vi "test_Multiple Static Single Channel Command Messages using Trigger and Padding.vi"(8 "error in (no error)":errorcluster, 11 "TestCase in":refnum<class "Common System Tests.lvclass">) -> (0 "error out":errorcluster, 3 "TestCase out":refnum<class "Common System Tests.lvclass">)   [LabVIEW 2018, in "Common System Tests.lvclass"]
uses:
  Common System Tests.lvclass
  <vilib>/addons/_JKI Toolkits/VI Tester/TestCase.llb/TestCase.lvclass
  <vilib>/NI VeriStand/Execution/Workspace/NI_VS Workspace ExecutionAPI.lvlib
  <vilib>/NI VeriStand/Execution/Workspace/NI VeriStand - Set Single Channel Value.vi
  <vilib>/NI VeriStand/Execution/Workspace/NI VeriStand - Get Multiple Channel Values.vi
  C:/Program Files (x86)/National Instruments/LabVIEW 2019/vi.lib/addons/_JKI Toolkits/VI Tester/TestCase.llb/TestCase.lvclass
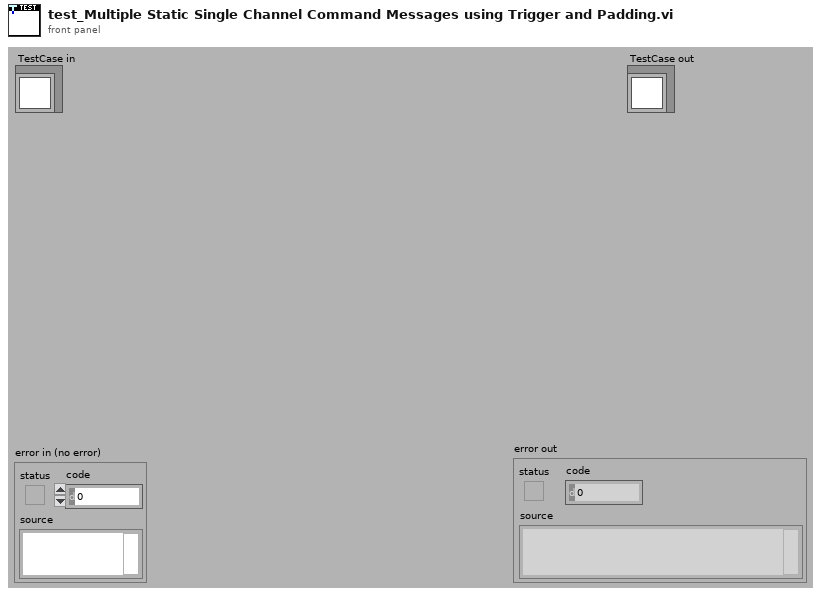
[diagram p1: front panel]
types:
  T1 = typedef "NI_VS Workspace ExecutionAPI.lvlib/WorkspaceAPI.ctl" = refnum<k24>
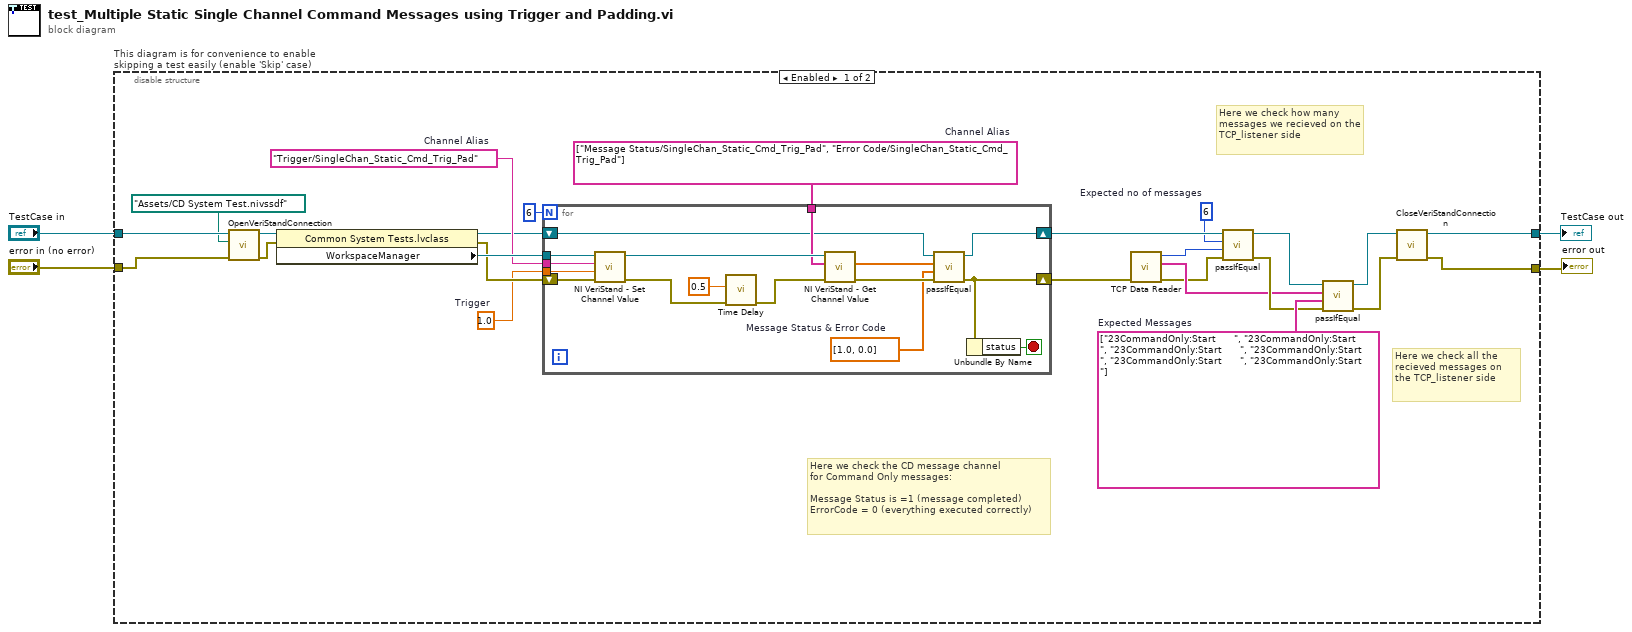
[diagram p0: block diagram]
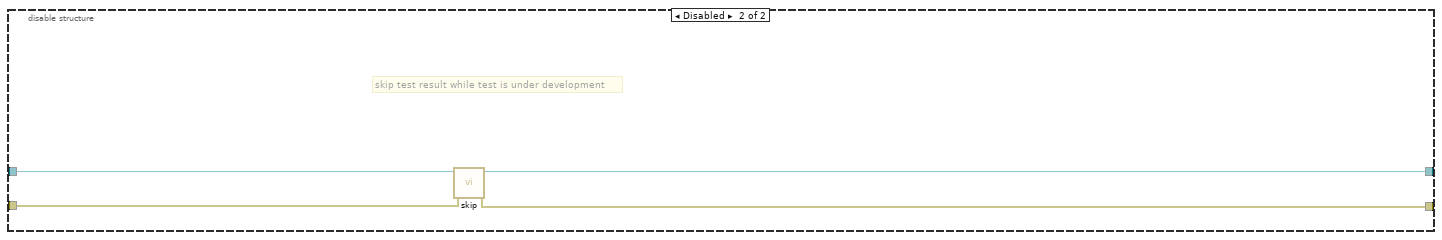
[diagram p2: hidden frame]
diagram:
  n1 = disable-structure "This diagram is for convenience to enable skipping a test easily (enable 'Skip' case)" shown="Enabled" {
    disable-tunnel: "TestCase in" -> [w27 w49]
    disable-tunnel: [w28 w47] -> w1
    disable-tunnel: [w29 w48] -> w3
    disable-tunnel: "error in (no error)" -> [w25 w46]
    frame Enabled {
      w11 = string[] ["23CommandOnly:Start      ", "23CommandOnly:Start      ", "23CommandOnly:Start      ", "23CommandOnly:Start      ", "23CommandOnly:Start      ", "23CommandOnly:Start      "]  # Expected Messages
      w13 = string[] ["Message Status/SingleChan_Static_Cmd_Trig_Pad", "Error Code/SingleChan_Static_Cmd_Trig_Pad"]  # Channel Alias
      w10 = 6  # Expected no of messages
      w19 = 1.0  # Trigger
      w20 = "Trigger/SingleChan_Static_Cmd_Trig_Pad"  # Channel Alias
      # "Here we check all the recieved messages on the TCP_listener side"
      # "Here we check how many messages we recieved on the TCP_listener side"
      # "Here we check the CD message channel\nfor Command Only messages:\n\nMessage Status is =1 (message completed)\nErrorCode = 0 (everything executed correctly)"
      n2 = call-dynamic "OpenVeriStandConnection.vi"("error in (no error)"=w25, "System Definition File"=path "Assets/CD System Test.nivssdf", "VeriStand Test Case in"=w27) -> ("error out"=w24:errorcluster, "VeriStand Test Case out"=w26:refnum<class "Common System Tests.lvclass">)  [unwired: 6 in, 1 out]
      n3 = property class="Common System Tests.lvclass"(reference=w26, error in=w24) -> (reference out=w17:refnum<class "Common System Tests.lvclass">, error out=w21:errorcluster, "WorkspaceManager"=w22:T1)
      n4 = for {
        N: 6 -> [_]
        tunnel: w22 -> [w45]
        tunnel: w20 -> [w43]
        tunnel: w19 -> [w42]
        shift-right: [w31] -> w5
        shift-left: w21 -> [w44]
        tunnel: w13 -> [w40]
        shift-right: [w35] -> w12
        shift-left: w17 -> [w36]
        stop <- w30 stop-if-true
        w32 = dbl[] [1.0, 0.0]  # Message Status & Error Code
        n5 = call-poly <vilib>:"NI VeriStand - Set Channel Value.vi"("error in (no error)"=w44, "Value"=w42, "Channel"=w43, "WorkspaceManager in"=w45) -> ("error out"=w38:errorcluster, "WorkspaceManager out"=w41:T1)  [unwired: 6 in]
        n6 = call "Time Delay"("error in (no error)"=w38, "Delay Time (s)"=0.5) -> ("error out"=w37:errorcluster)  [unwired: 9 in]
        n7 = call-poly <vilib>:"NI VeriStand - Get Channel Value.vi"("error in (no error)"=w37, "Channels"=w40, "WorkspaceManager in"=w41) -> ("error out"=w34:errorcluster, "Values"=w33:dbl[])  [unwired: 6 in, 1 out]
        n8 = call-dynamic "passIfEqual.vi"("error in (no error)"=w34, "y"=w32, "x"=w33, "TestCase in"=w36) -> ("error out"=w31:errorcluster, "TestCase out"=w35:refnum<class "Common System Tests.lvclass">)  [unwired: 6 in]
        n9 = Unbundle By Name(w31) -> ("status"=w30:bool)
      }
      n10 = call "TCP Data Reader.vi"("error in (no error)"=w5) -> ("error out"=w6:errorcluster, "Recieved Messages"=w7:string[], "No of messages"=w8:i32)  [unwired: 8 in]
      n11 = call-dynamic "passIfEqual.vi"("error in (no error)"=w6, "y"=w8, "x"=w10, "TestCase in"=w12) -> ("error out"=w9:errorcluster, "TestCase out"=w16:refnum<class "Common System Tests.lvclass">)  [unwired: 6 in]
      n12 = call-dynamic "passIfEqual.vi"("error in (no error)"=w9, "y"=w11, "x"=w7, "TestCase in"=w16) -> ("error out"=w14:errorcluster, "TestCase out"=w15:refnum<class "Common System Tests.lvclass">)  [unwired: 6 in]
      n13 = call-dynamic "CloseVeriStandConnection.vi"("error in (no error)"=w14, "VeriStand Test Case in"=w15) -> ("error out"=w29:errorcluster, "VeriStand Test Case out"=w28:refnum<class "Common System Tests.lvclass">)  [unwired: 8 in]
    }
    frame Disabled {
      # "skip test result while test is under development"
      n14 = call <vilib>:"skip.vi"("error in (no error)"=w46, "TestCase in"=w49) -> ("error out"=w48:errorcluster, "TestCase out"=w47:refnum<class "Common System Tests.lvclass">)  [unwired: 8 in]
    }
  }
  "error out" <- w3
  "TestCase out" <- w1
